vi "Unified Leaf.vi"(6 "Alias":string, 7 "Actor in":refnum<class "Actor.lvclass">) -> (0 "Error out":errorcluster, 2 "Unified Leaf":bool)   [LabVIEW 2020, in "jettl.lvlib" / "Read Child Attributes.lvlib"]
uses:
  Read Child Attributes.lvlib
  jettl.lvlib
  Actor/Actor.lvclass
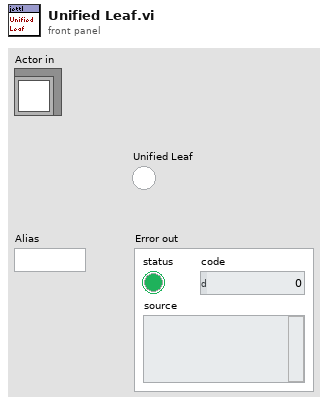
[diagram p1: front panel]
types:
  T1 = typedef "jettl.lvlib/Attributes.ctl" = cluster{"Unified Msgs":T2, "Unified Leaf":bool, "Edge Actors":refnum<class "Actor.lvclass">[], "Core Actors":refnum<class "Actor.lvclass">[], "Root":bool, "Alias":string, "UID":i32, "Transport":refnum<class "Transport.lvclass">, "This VI":refnum<vi>, "Attributes Metadata":refnum<class "Attributes Metadata.lvclass">, "Post-Setup Actors":refnum<class "Actor.lvclass">[]}
  T2 = typedef "jettl.lvlib/Msgs.ctl" = set{refnum<class "Msg.lvclass">}
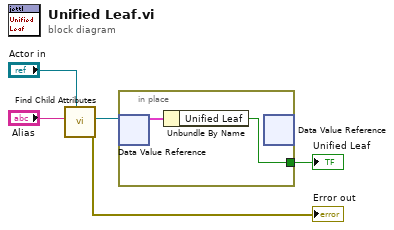
[diagram p0: block diagram]
diagram:
  n1 = call "Find Child Attributes.vi"("Actor in"="Actor in", "Alias"="Alias") -> ("Error out"=→"Error out":errorcluster, "Child Attributes"=w2:refnum<data-value>)  [unwired: 8 in]
  n2 = in-place {
    in-place-border: [w6] -> w1
    n3 = in-place-dvr #1(w2) -> (w7:T1)  [unwired: 1 out]
    n4 = Unbundle By Name(w7) -> ("Unified Leaf"=w6:bool)
    n5 = in-place-dvr #1() -> ()  [unwired: 1 in, 2 out]
  }
  "Unified Leaf" <- w1
